vi "Button Position based on Message dialog Box.vi"(0 "Pop-up Type":T1(ring), 1 "Message Width":u32=500, 2 "Message Left":u32=500, 3 "Button 1 Width":u32=500, 4 "Button 2 Width":u32=500, 5 "error in (no error)":errorcluster) -> (14 "Button 1 Left":u32, 15 "Button 2 Left":u32, 16 "Button Visible":bool, 19 "error out":errorcluster)   [LabVIEW 2019, in "ZenGage v3.0 UI.lvclass"]
uses:
  ZenGage v3.0 UI.lvclass
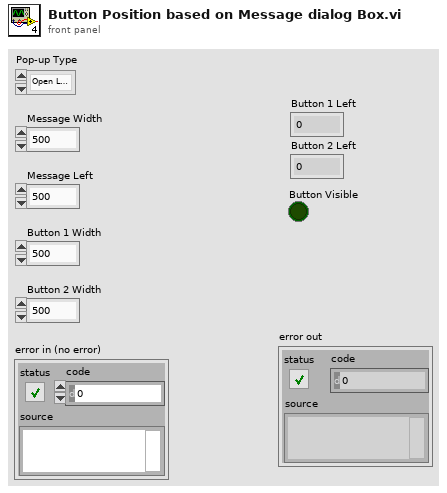
[diagram p1: front panel]
types:
  T1 = enum16{"Open Logo Display", "Close Logo Display", "Open Loading Bar", "Close Loading Bar", "Open Alert Display", "Close Alert Display", "One button dialog box", "Two button dialog box", "User Authentication"}
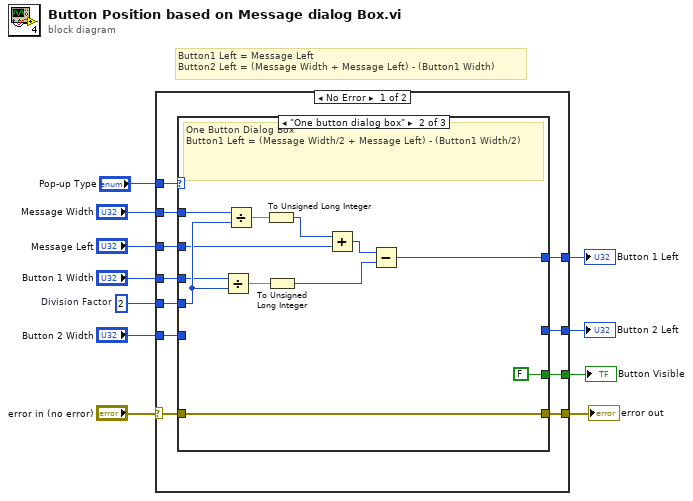
[diagram p0: block diagram]
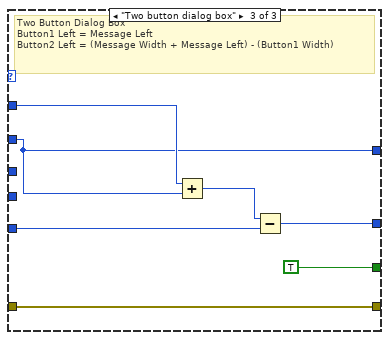
[diagram p3: hidden frame]
diagram:
  w11 = u32 2  # Division Factor
  # "Button1 Left = Message Left\nButton2 Left = (Message Width + Message Left) - (Button1 Width)"
  n1 = case shown="No Error" "error in (no error)" {
    selector: "error in (no error)" -> [w12 w43]
    tunnel: w11 -> [w22 _]
    tunnel: "Message Width" -> [w21 _]
    tunnel: "Button 1 Width" -> [w20 _]
    tunnel: [w19 _] -> w8
    tunnel: "Message Left" -> [w18 _]
    tunnel: "Button 2 Width" -> [w17 _]
    tunnel: [w16 _] -> w5
    tunnel: "Pop-up Type" -> [w15 _]
    tunnel: [w14 _] -> w3
    tunnel: [w13 w43] -> w2
    frame No Error {
      n2 = case shown="\"One button dialog box\"" w15 {
        tunnel: w22 -> [_ w32 _]
        tunnel: w21 -> [_ w33 w42]
        tunnel: w20 -> [_ w31 _]
        tunnel: [_ w26 w41] -> w19
        tunnel: w18 -> [_ w29 w41]
        tunnel: w17 -> [_ _ w39]
        tunnel: [_ _ w38] -> w16
        tunnel: [_ FALSE TRUE] -> w14
        tunnel: [w23 w24 w36] -> w13
        tunnel: w12 -> [w23 w24 w36]
        frame Default {
        }
        frame "One button dialog box" {
          # "One Button Dialog Box\nButton1 Left = (Message Width/2 + Message Left) - (Button1 Width/2)"
          n3 = Divide(x=w31, y=w32) -> (x/y=w30:dbl)
          n4 = Divide(x=w33, y=w32) -> (x/y=w35:dbl)
          n5 = To Unsigned Long Integer(number=w35) -> (unsigned 32bit integer=w34:u32)
          n6 = To Unsigned Long Integer(number=w30) -> (unsigned 32bit integer=w27:u32)
          n7 = Add(x=w34, y=w29) -> (x+y=w28:u32)
          n8 = Subtract(x=w28, y=w27) -> (x-y=w26:u32)
        }
        frame "Two button dialog box" {
          # "Two Button Dialog Box\nButton1 Left = Message Left\nButton2 Left = (Message Width + Message Left) - (Button1 Width)"
          n9 = Add(x=w42, y=w41) -> (x+y=w40:u32)
          n10 = Subtract(x=w40, y=w39) -> (x-y=w38:u32)
        }
      }
    }
    frame Error {
    }
  }
  "Button 1 Left" <- w8
  "Button 2 Left" <- w5
  "Button Visible" <- w3
  "error out" <- w2
